vi "Load Async.vi"(8 "error in (no error)":errorcluster, 9 "Channels":u32, 10 "Path":string, 11 "Channel in":refnum<data-value>) -> (0 "error out":errorcluster, 3 "Channel out":refnum<data-value>)   [LabVIEW 2020, in "G-Audio.lvlib" / "Channel.lvclass"]
uses:
  Channel.lvclass
  Controls/Channel State.ctl
  Channel.lvclass/Channel.ctl
  Mixer/Controls/Mixer Audio Data Type.ctl
  88edfe70-fc9c-4621-9b1b-9ed93909f707.vi
  78e39600-8aee-4b0a-9192-f4b43d78cbe5.vi/a9b40114-c599-493c-b53b-ddbd5bd76bb4.vi
  78e39600-8aee-4b0a-9192-f4b43d78cbe5.vi/2f1d6506-1e95-426b-9767-108adecdc3c4.vi
  78e39600-8aee-4b0a-9192-f4b43d78cbe5.vi/e1e9c27a-47b3-4558-a963-a0614bd48cc9.vi
  Private/Result To Error.vi
  Private/Get Basic Audio File Info.vi
  9b2e347b-653f-4c08-ac62-7d080a165944.vi/779dfdfd-1b42-4cf4-8001-66d3dd167625.vi
  9b2e347b-653f-4c08-ac62-7d080a165944.vi/55d550d4-9624-414e-aebd-6e02b5081896.vi
  Private/Audio File Refnum To Value.vi
  78e39600-8aee-4b0a-9192-f4b43d78cbe5.vi/a9b40114-c599-493c-b53b-ddbd5bd76bb4.vi/4b7b629c-2e91-4160-9820-a26af8f6e677.vi
  78e39600-8aee-4b0a-9192-f4b43d78cbe5.vi/2f1d6506-1e95-426b-9767-108adecdc3c4.vi/4b7b629c-2e91-4160-9820-a26af8f6e677.vi
  9b2e347b-653f-4c08-ac62-7d080a165944.vi/55d550d4-9624-414e-aebd-6e02b5081896.vi/4b7b629c-2e91-4160-9820-a26af8f6e677.vi
  Audio Files/Polymorphic VIs/Get Audio File Info (UTF-8).vi
  Audio Files/Polymorphic VIs/Open Audio File Read (UTF-8).vi
  <vilib>/Utility/Data Type/Get Numeric Information.vi
  <vilib>/Utility/error.llb/Error Cluster From Error Code.vi
  G-Audio.lvlib
  Mixer/Mixer.lvclass
  43543127-e5ae-408e-8e9d-53e21a79ca6d.vi
  8d24f717-3bac-45af-9960-9a5be7c21528.vi
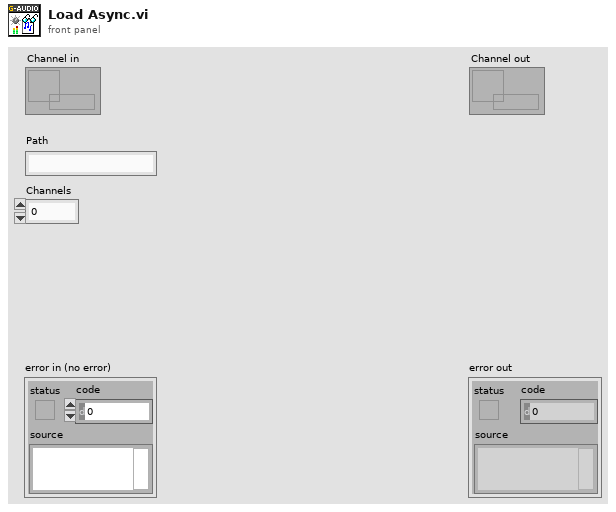
[diagram p1: front panel]
types:
  T1 = typedef "G-Audio.lvlib/Channel.lvclass/Channel State.ctl" = enum16{"Empty", "Error", "Loading", "Loaded", "Stopped", "Paused", "Playing", "Retrigger"}
  T2 = typedef "G-Audio.lvlib/Mixer.lvclass/Mixer Audio Data Type.ctl" = i16[][]
  T3 = typedef "G-Audio.lvlib/Audio File Refnum.ctl" = refnum<file>
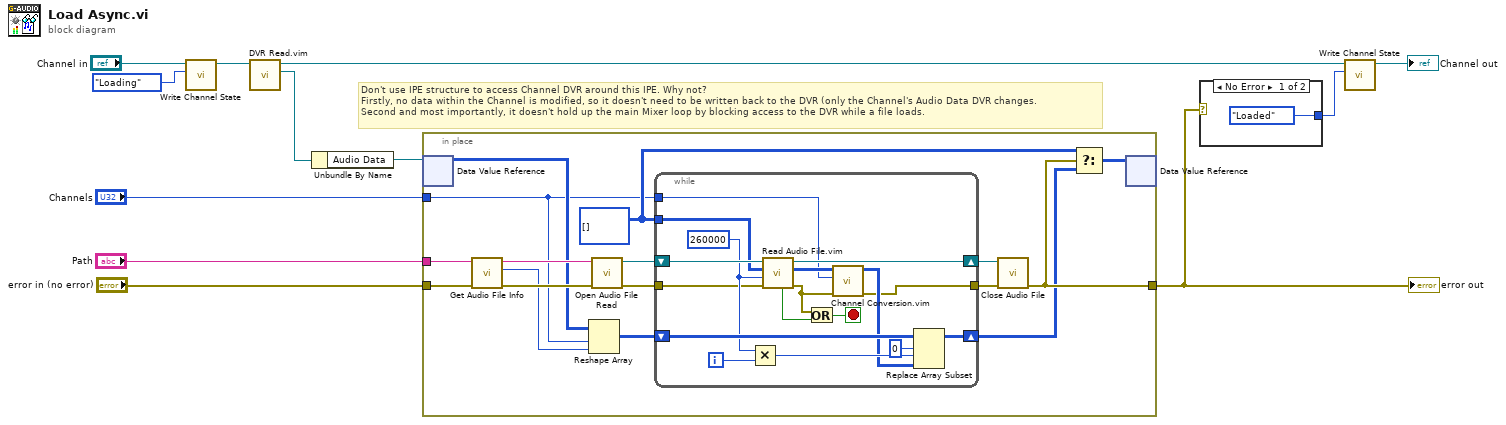
[diagram p0: block diagram]
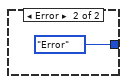
[diagram p2: hidden frame]
diagram:
  # "Don't use IPE structure to access Channel DVR around this IPE. Why not?\nFirstly, no data within the Channel is modified, so it doesn't need to be written back to the DVR (only the Channel's Audio Data DVR changes.\nSecond and most importantly, it doesn't hold up the main Mixer loop by blocking access to the DVR while a file loads."
  n1 = call "Write Channel State.vi"("State"=Channel_State."Loading", "Channel in"="Channel in") -> ("Channel out"=w3:refnum<data-value>)  [unwired: 8 in, 1 out]
  n2 = call "DVR Read.vim"("DVR In"=w3) -> ("Data"=w4:refnum<class "Channel.lvclass">, "DVR Out"=w2:refnum<data-value>)  [unwired: 9 in]
  n3 = Unbundle By Name(w4) -> ("Audio Data"=w5:refnum<data-value>)
  n4 = in-place {
    in-place-border: "Path" -> [w22]
    in-place-border: "error in (no error)" -> [w21]
    in-place-border: [w17] -> w8
    in-place-border: "Channels" -> [w13]
    w14 = T2 [] ("Audio Data Type")
    n5 = in-place-dvr #1(w5) -> (w20:T2)  [unwired: 1 out]
    n6 = call-poly "Get Audio File Info.vi"("error in (no error)"=w21, "Path In"=w22) -> ("error out"=w27:errorcluster, "PCM Frame Length"=w19:u64, "Path Out"=w28:string)  [unwired: 5 in, 2 out]
    n7 = Reshape Array(w20, w13, w19) -> (w18:T2)
    n8 = call-poly "Open Audio File Read.vi"("error in (no error)"=w27, "Path"=w28) -> ("error out"=w23:errorcluster, "Audio File Refnum"=w26:T3)  [unwired: 8 in]
    n9 = while {
      shift-right: [w42] -> w16
      shift-left: w18 -> [w38]
      shift-right: [w41] -> w25
      shift-left: w26 -> [w37]
      tunnel: w14 -> [w36]
      tunnel: [w30] -> w24
      tunnel: w23 -> [w34]
      tunnel: w13 -> [w29]
      i -> [w44]
      stop <- w39 stop-if-true
      w35 = u64 260000 ("Frames To Read")
      n10 = Multiply(x=w35, y=w44) -> (x*y=w43:u64)
      n11 = call "Read Audio File.vim"("error in (no error)"=w34, "Frames To Read"=w35, "Data Format"=w36, "Audio File Refnum In"=w37) -> ("error out"=w31:errorcluster, "Audio Data"=w33:T2, "Audio File Refnum Out"=w41:T3, "End of File?"=w40:bool)  [unwired: 3 in, 1 out]
      n12 = Or(x=w31, y=w40) -> (x .or. y?=w39:bool)
      n13 = call "Channel Conversion.vim"("error in (no error)"=w31, "Channels"=w29, "Audio Data in"=w33) -> ("error out"=w30:errorcluster, "Audio Data out"=w32:T2)  [unwired: 7 in]
      n14 = Replace Array Subset(array=w38, new element=w32, index (row)=0 ("disabled index (row)"), index (col)=w43) -> (w42:T2)
    }
    n15 = call "Close Audio File.vi"("error in (no error)"=w24, "Audio File Refnum In"=w25) -> ("error out"=w17:errorcluster)  [unwired: 9 in]
    n16 = Select(t=w14, s=w17, f=w16) -> (s? t:f=w15:T2)
    n17 = in-place-dvr #1(w15) -> ()  [unwired: 2 out]
  }
  "error out" <- w8
  n18 = case shown="No Error" w8 {
    tunnel: [Channel_State."Loaded" ("State") Channel_State."Error" ("State")] -> w12
    frame No Error {
    }
    frame Error {
    }
  }
  n19 = call "Write Channel State.vi"("State"=w12, "Channel in"=w2) -> ("Channel out"=→"Channel out":refnum<data-value>)  [unwired: 8 in, 1 out]
